vi "Facade.vi"(0 "Data In":T5, 2 "Display State In":T3={"Precision"=6, "Format"=6, "Formula"=""} {"Format" items=["Decimal"=0, "Scientific"=1, "Hexadecimal"=5]}, 3 "Container State":T4) -> (6 "Data Out":T5, 7 "Display State Out":T3={"Precision"=6, "Format"=6, "Formula"=""} {"Format" items=["Decimal"=0, "Scientific"=1, "Hexadecimal"=5]}, 8 "Action":T2)   [LabVIEW 2013, in "Calculator XControl.xctl"]
doc: "This VI defines the appearance and behavior of the Calculator XControl. The front panel of the Facade VI defines the appearance of the XControl. The block diagram of the Facade VI describes the behavior of the XControl, using an Event Structure to define responses to various events that can occur on the XControl."
uses:
  Calculator XControl.xctl
  Data.ctl
  <vilib>/_xctls/Container State.ctl
  State.ctl
  Controls/Format.ctl
  <vilib>/_xctls/Action.ctl
  <vilib>/event_ctls.llb/eventvkey.ctl
  <vilib>/_xctls/XControlSupport.lvlib
panel:
  out "Output":string
  in  "Backspace":bool
  in  "(":bool
  in  ")":bool
  in  "^":bool
  in  "E":bool
  in  "Tab Control":enum32{"Func", "Symbol"}(tab)
  in  "Cot":bool
  in  "Csc":bool
  in  "Sec":bool
  in  "e^":bool
  in  "tanh":bool
  in  "cosh":bool
  in  "sinh":bool
  in  "log":bool
  in  "ln":bool
  in  "Tan":bool
  in  "Cos":bool
  in  "Sin":bool
  in  "NA":bool
  in  "R":bool
  in  "c":bool
  in  "exp":bool
  in  "pi":bool
  in  "Answer":bool
  in  "Clear":bool
  in  "Precision":u8=6
  in  "Format":T1 items=["Decimal"=0, "Scientific"=1, "Hexadecimal"=5]
  in  "Equals":bool
  in  "Nine":bool
  in  "Eight":bool
  in  "Seven":bool
  in  "Six":bool
  in  "Five":bool
  in  "Four":bool
  in  "Decimal":bool
  in  "Three":bool
  in  "Two":bool
  in  "Zero":bool
  in  "One":bool
  in  "Divide":bool
  in  "Multiply":bool
  in  "Minus":bool
  in  "Plus":bool
  in  "Formula":string
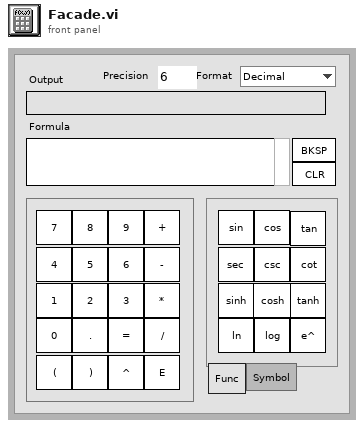
[diagram p1: front panel]
types:
  T1 = typedef "Calculator XControl.xctl/Format.ctl" = u16
  T2 = typedef "XControlSupport.lvlib/Action.ctl" = cluster{"Data Changed?":bool, "State Changed?":bool, "Action Name":string}
  T3 = typedef "Calculator XControl.xctl/State.ctl" = cluster{"Precision":u8, "Format":T1, "Formula":string}
  T4 = typedef "XControlSupport.lvlib/Container State.ctl" = cluster{"Indicator?":bool, "Run Mode?":bool, " Refnum":refnum<vi>}
  T5 = typedef "Calculator XControl.xctl/Data.ctl" = dbl
  T6 = typedef "eventvkey.ctl" = enum16{"ASCII", "Enter", "Return", "Shift", "Ctrl", "Alt", "Cmd", "Opt", "Caps", "NumLock", "Clear", "Break", "Up", "Down", "Left", "Right", "Insert", "Delete", "Home", "End", "PageUp", "PageDown", "Escape", "Help", "Pause", "ScrollLock", "F1", "F2", "F3", "F4", "F5", "F6", "F7", "F8", "F9", "F10", "F11", "F12", "F13", "F14", "F15", "F16", "F17", "F18", "F19", "F20", "F21", "F22", "F23", "F24", "Play", "VolumeUp", "VolumeDown", "Mute", "Two Byte Char"}
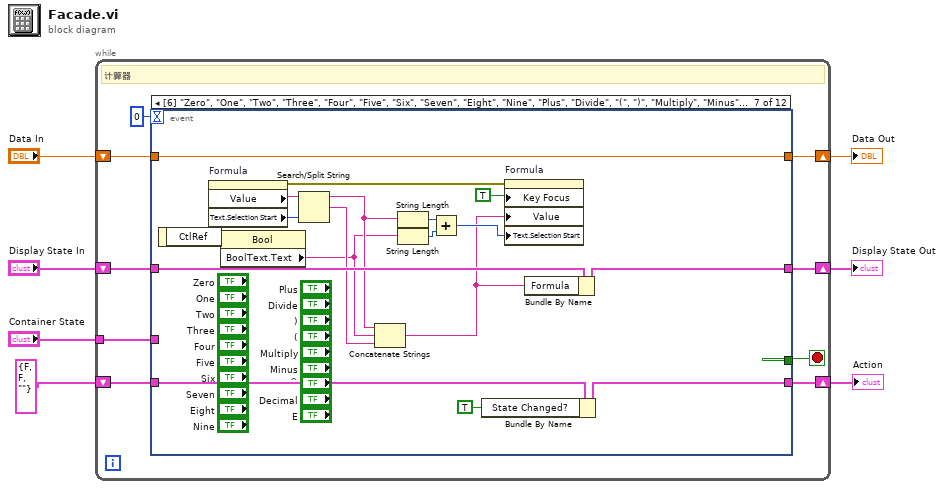
[diagram p0: block diagram]
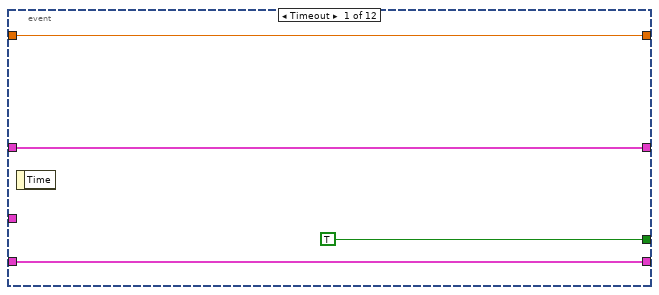
[diagram p2: hidden frame]
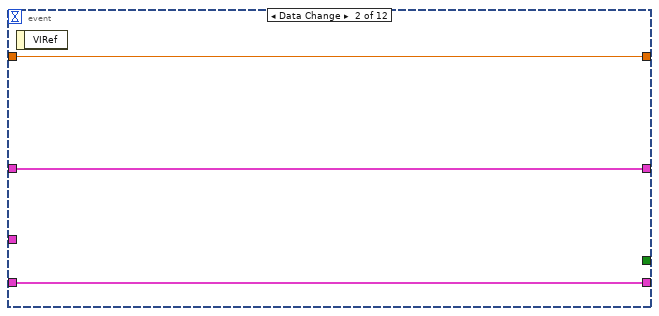
[diagram p3: hidden frame]
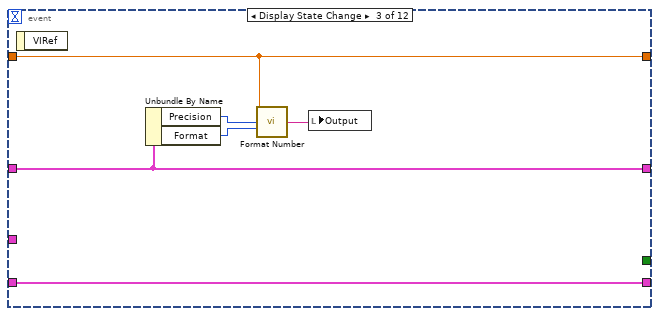
[diagram p4: hidden frame]
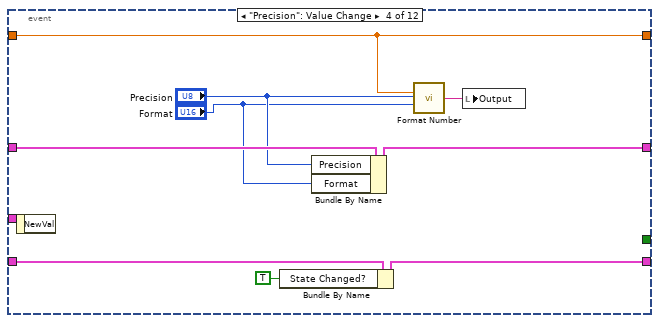
[diagram p5: hidden frame]
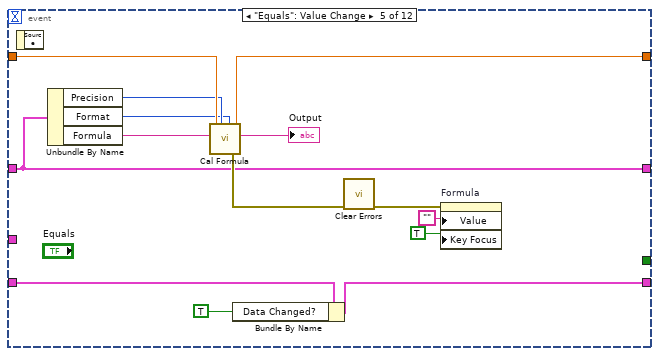
[diagram p6: hidden frame]
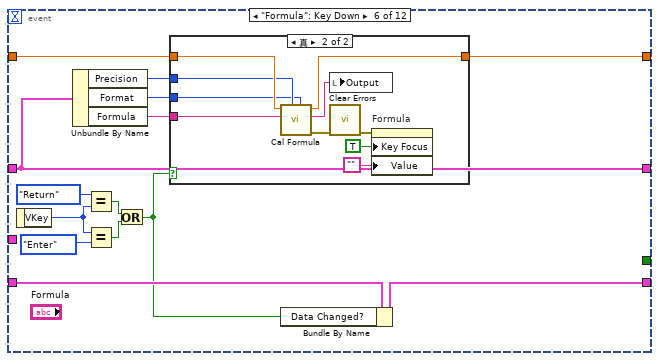
[diagram p7: hidden frame]
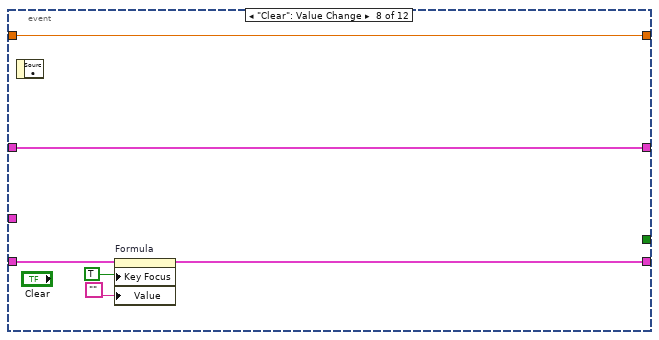
[diagram p9: hidden frame]
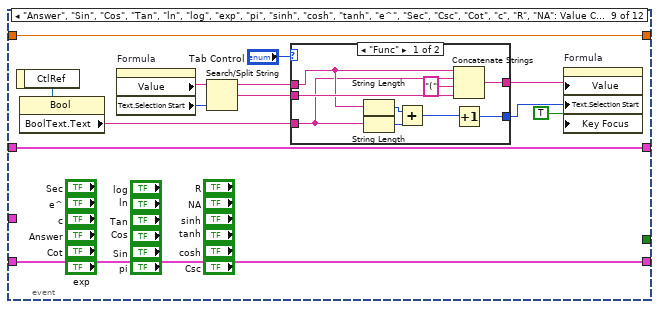
[diagram p10: hidden frame]
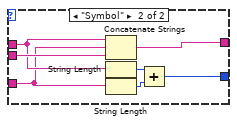
[diagram p11: hidden frame]
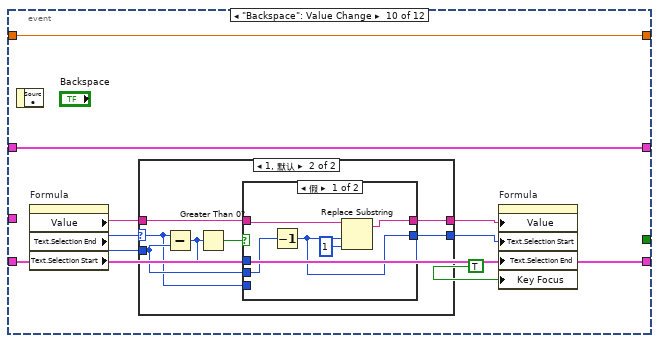
[diagram p12: hidden frame]
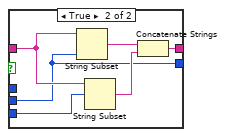
[diagram p14: hidden frame]
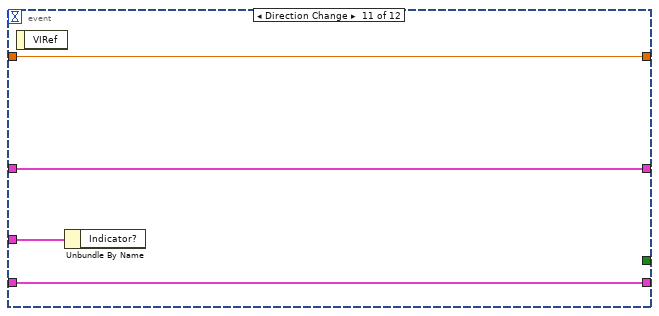
[diagram p15: hidden frame]
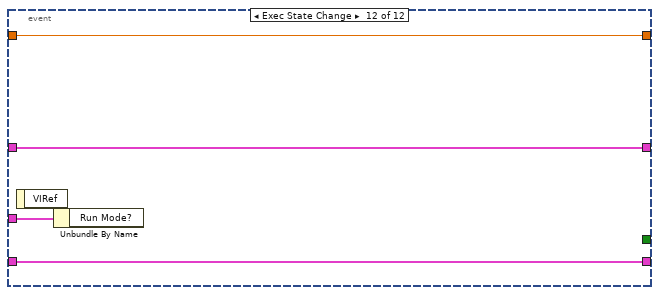
[diagram p16: hidden frame]
diagram:
  n1 = while {
    shift-right: [w15] -> w4
    shift-left: "Display State In" -> [w16]
    tunnel: "Container State" -> [w12]
    shift-right: [w10] -> w7
    shift-left: "Data In" -> [w11]
    shift-right: [w8] -> w2
    shift-left: T2 {"Data Changed?"=FALSE, "State Changed?"=FALSE, "Action Name"=""} ("Action") -> [w9]
    stop <- w14 stop-if-true
    # "计算器"
    n2 = event shown="[6] \"Zero\", \"One\", \"Two\", \"Three\", \"Four\", \"Five\", \"Six\", \"Seven\", \"Eight\", \"Nine\", \"Plus\", \"Divide\", \"(\", \")\", \"Multiply\", \"Minus\", \"^\", \"Decimal\", \"E\": 值改变" {
      selector: _ -> [_ _ _ _ _ _ _ _ _ _ _ _]
      dyn-events: _ -> [_ _ _ _ _ _ _ _ _ _ _ _]
      timeout: 0 -> [_ _ _ _ _ _ _ _ _ _ _ _]
      tunnel: w16 -> [w18 w23 w26 w38 w43 w56 w94 w100 w112 w137 w161 w165]
      tunnel: [w18 w23 w26 w34 w43 w56 w81 w100 w112 w137 w161 w165] -> w15
      tunnel: [TRUE _ _ _ _ _ _ _ _ _ _ _] -> w14
      tunnel: w12 -> [_ _ _ _ _ _ _ _ _ _ w162 w166]
      tunnel: w11 -> [w17 w21 w28 w36 w46 w66 w93 w98 w113 w138 w160 w164]
      tunnel: [w17 w21 w28 w36 w45 w63 w93 w98 w113 w138 w160 w164] -> w10
      tunnel: [w19 w22 w29 w31 w51 w64 w79 w99 w111 w136 w159 w163] -> w8
      tunnel: w9 -> [w19 w22 w29 w37 w52 w65 w95 w99 w111 w136 w159 w163]
      event Timeout {
        n3 = event-data() -> ()  [unwired: 1 in, 1 out]
      }
      event Data Change {
        n4 = event-data() -> ()  [unwired: 1 in, 1 out]
      }
      event Display State Change {
        n5 = event-data() -> ()  [unwired: 1 in, 1 out]
        n6 = Unbundle By Name(w26) -> ("Precision"=w25:u8, "Format"=w24:T1)
        n7 = call "Format Number.vi"("Data"=w28, "precision (6)"=w25, "Format"=w24) -> ("Numeric String"=w27:string)  [unwired: 12 in]
        n8 = local write "Output"(w27) -> ()
      }
      event "Precision": Value Change {
        n9 = event-data() -> ()  [unwired: 1 in, 1 out]
        n10 = Bundle By Name(cluster=w37, "State Changed?"=TRUE) -> (w31:T2)
        n11 = Bundle By Name(cluster=w38, "Precision"="Precision", "Format"="Format") -> (w34:T3)
        n12 = call "Format Number.vi"("Data"=w36, "precision (6)"="Precision", "Format"="Format") -> ("Numeric String"=w35:string)  [unwired: 12 in]
        n13 = local write "Output"(w35) -> ()
      }
      event "Equals": Value Change {
        n14 = event-data() -> ()  [unwired: 1 in, 1 out]
        n15 = Unbundle By Name(w43) -> ("Precision"=w42:u8, "Format"=w41:T1, "Formula"=w40:string)
        n16 = call "Cal Formula.vi"("Format"=w41, "precision (6)"=w42, "Formula In"=w40, "Data In"=w46) -> ("error out"=w44:errorcluster, "Numeric String"=→"Output":string, "Data Out"=w45:dbl)  [unwired: 5 in]
        n17 = Bundle By Name(cluster=w52, "Data Changed?"=TRUE) -> (w51:T2)
        n18 = call <vilib>:"Clear Errors.vi"("error in (no error)"=w44) -> ("error out"=w47:errorcluster)  [unwired: 6 in]
        n19 = property on="Formula" class="Str"(error in=w47, "Value"="", "Key Focus"=TRUE) -> ()  [unwired: 1 in, 2 out]
      }
      event "Formula": Key Down {
        n20 = event-data() -> ("VKey"=w61:T6)  [unwired: 1 in]
        n21 = Unbundle By Name(w56) -> ("Precision"=w55:u8, "Format"=w54:T1, "Formula"=w53:string)
        n22 = Equal?(x=eventvkey."Return" ("y"), y=w61) -> (x = y?=w59:bool)
        n23 = Equal?(x=w61, y=eventvkey."Enter") -> (x = y?=w58:bool)
        n24 = Or(x=w59, y=w58) -> (x .or. y?=w57:bool)
        n25 = case shown="真" w57 {
          tunnel: w66 -> [w67 w74]
          tunnel: [w67 w73] -> w63
          tunnel: w55 -> [_ w70]
          tunnel: w54 -> [_ w69]
          tunnel: w53 -> [_ w68]
          frame False {
          }
          frame True {
            n26 = call "Cal Formula.vi"("Format"=w69, "precision (6)"=w70, "Formula In"=w68, "Data In"=w74) -> ("error out"=w71:errorcluster, "Numeric String"=w72:string, "Data Out"=w73:dbl)  [unwired: 5 in]
            n27 = local write "Output"(w72) -> ()
            n28 = call <vilib>:"Clear Errors.vi"("error in (no error)"=w71) -> ("error out"=w75:errorcluster)  [unwired: 6 in]
            n29 = property on="Formula" class="Str"(error in=w75, "Key Focus"=TRUE, "Value"="") -> ()  [unwired: 1 in, 2 out]
          }
        }
        n30 = Bundle By Name(cluster=w65, "Data Changed?"=w57) -> (w64:T2)
      }
      event "Zero", "One", "Two", "Three", "Four", "Five", "Six", "Seven", "Eight", "Nine", "Plus", "Divide", "(", ")", "Multiply", "Minus", "^", "Decimal", "E": Value Change {
        n31 = event-data() -> ("CtlRef"=w83:refnum<vi>)  [unwired: 1 in]
        n32 = property on="Formula" class="Str"() -> (error out=w89:errorcluster, "Value"=w92:string, "Text.Selection Start"=w91:u32)  [unwired: 2 in, 1 out]
        n33 = property class="Bool"(reference=w83) -> ("BoolText.Text"=w82:string)  [unwired: 1 in, 2 out]
        n34 = Search/Split String(string=w92, offset (0)=w91) -> (substring before match=w87:string, match + rest of string=w90:string)  [unwired: 1 in, 1 out]
        n35 = Concatenate Strings(w87, w82, w90) -> (w80:string)
        n36 = String Length(string=w87) -> (length=w86:i32)
        n37 = String Length(string=w82) -> (length=w85:i32)
        n38 = Add(x=w86, y=w85) -> (x+y=w84:i32)
        n39 = Bundle By Name(cluster=w95, "State Changed?"=TRUE) -> (w79:T2)
        n40 = property on="Formula" class="Str"(error in=w89, "Key Focus"=TRUE, "Value"=w80, "Text.Selection Start"=w84) -> ()  [unwired: 1 in, 2 out]
        n41 = Bundle By Name(cluster=w94, "Formula"=w80) -> (w81:T3)
      }
      event "Clear": Value Change {
        n42 = event-data() -> ()  [unwired: 1 in, 1 out]
        n43 = property on="Formula" class="Str"("Key Focus"=TRUE, "Value"="") -> ()  [unwired: 2 in, 2 out]
      }
      event "Answer", "Sin", "Cos", "Tan", "ln", "log", "exp", "pi", "sinh", "cosh", "tanh", "e^", "Sec", "Csc", "Cot", "c", "R", "NA": Value Change {
        n44 = event-data() -> ("CtlRef"=w110:refnum<vi>)  [unwired: 1 in]
        n45 = property class="Bool"(reference=w110) -> ("BoolText.Text"=w102:string)  [unwired: 1 in, 2 out]
        n46 = property on="Formula" class="Str"() -> ("Value"=w109:string, "Text.Selection Start"=w108:u32)  [unwired: 2 in, 2 out]
        n47 = Search/Split String(string=w109, offset (0)=w108) -> (substring before match=w107:string, match + rest of string=w106:string)  [unwired: 1 in, 1 out]
        n48 = case shown="\"Func\"" "Tab Control" {
          tunnel: [w121 w129] -> w104
          tunnel: w107 -> [w119 w125]
          tunnel: w106 -> [w120 w128]
          tunnel: [w115 w124] -> w103
          tunnel: w102 -> [w114 w123]
          frame "Func" {
            n49 = String Length(string=w119) -> (length=w117:i32)
            n50 = String Length(string=w114) -> (length=w118:i32)
            n51 = Add(x=w117, y=w118) -> (x+y=w116:i32)
            n52 = Concatenate Strings(w119, w114, "(" ("string"), w120) -> (w121:string)
            n53 = Increment(x=w116) -> (x+1=w115:i32)
          }
          frame "Symbol" {
            n54 = Concatenate Strings(w125, w123, w128) -> (w129:string)
            n55 = String Length(string=w125) -> (length=w126:i32)
            n56 = String Length(string=w123) -> (length=w127:i32)
            n57 = Add(x=w126, y=w127) -> (x+y=w124:i32)
          }
        }
        n58 = property on="Formula" class="Str"("Value"=w104, "Text.Selection Start"=w103, "Key Focus"=TRUE) -> ()  [unwired: 2 in, 2 out]
      }
      event "Backspace": Value Change {
        n59 = event-data() -> ()  [unwired: 1 in, 1 out]
        n60 = property on="Formula" class="Str"() -> ("Value"=w134:string, "Text.Selection End"=w130:u32, "Text.Selection Start"=w135:u32)  [unwired: 2 in, 2 out]
        n61 = case shown="1, 默认" w130 {
          selector: w130 -> [w139 w141]
          tunnel: w135 -> [_ w146]
          tunnel: w134 -> [w140 w145]
          tunnel: [w140 w143] -> w132
          tunnel: [w139 w142] -> w131
          frame 0 {
          }
          frame 1, Default {
            n62 = Subtract(x=w141, y=w146) -> (x-y=w144:u32)
            n63 = Greater Than 0?(x=w144) -> (x > 0?=w147:bool)
            n64 = case shown="假" w147 {
              tunnel: w146 -> [w149 w153]
              tunnel: w141 -> [_ w157]
              tunnel: w145 -> [w152 w158]
              tunnel: w144 -> [_ _]
              tunnel: [w150 w154] -> w143
              tunnel: [w148 w153] -> w142
              frame False {
                n65 = Decrement(x=w149) -> (x-1=w148:u32)
                n66 = Replace Substring(2:1 ("length (len. of substring)"), 3:w148, 5:w152) -> (1:w150:string)  [unwired: 1 in, 1 out]
              }
              frame True {
                n67 = String Subset(string=w158, length (rest)=w153) -> (substring=w156:string)  [unwired: 1 in]
                n68 = String Subset(string=w158, offset (0)=w157) -> (substring=w155:string)  [unwired: 1 in]
                n69 = Concatenate Strings(w156, w155) -> (w154:string)
              }
            }
          }
        }
        n70 = property on="Formula" class="Str"("Value"=w132, "Text.Selection Start"=w131, "Text.Selection End"=w131, "Key Focus"=TRUE) -> ()  [unwired: 2 in, 2 out]
      }
      event Direction Change {
        n71 = event-data() -> ()  [unwired: 1 in, 1 out]
        n72 = Unbundle By Name(w162) -> ()  [unwired: 1 out]
      }
      event Exec State Change {
        n73 = event-data() -> ()  [unwired: 1 in, 1 out]
        n74 = Unbundle By Name(w166) -> ()  [unwired: 1 out]
      }
    }
  }
  "Display State Out" <- w4
  "Data Out" <- w7
  "Action" <- w2
